vi "HEX string to ASCII string.vi"(9 "String In":string) -> (1 "String Out":string)   [LabVIEW 2014]
panel:
  # "Convert a string of hex ASCII values to an ASCII string"
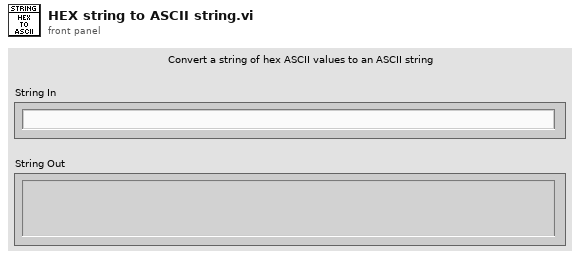
[diagram p1: front panel]
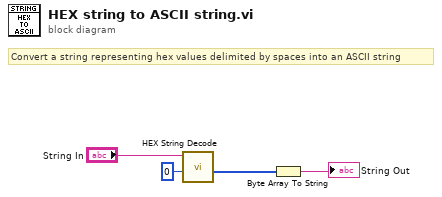
[diagram p0: block diagram]
diagram:
  # "Convert a string representing hex values delimited by spaces into an ASCII string"
  n1 = call "HEX String Decode.vi"("Values To Decode"=u16 0, "String In"="String In") -> ("Array"=w2:u32[])  [unwired: 7 in, 1 out]
  n2 = Byte Array To String(unsigned byte array=w2) -> (string=→"String Out":string)
